vi "Write.vi"(5 "Maximum File Size (Bytes)":i64, 6 "Options":T1={"Delete All Excessive"=FALSE, "Delimiter"=",", "Enable Calendar Tree"=TRUE, "File Extension"="csv", "Time Stamp Format"="%Y%m%dT%H%M%S%3u"}, 7 "Maximum File Count":i32, 8 "Error In":errorcluster, 9 "Messages":T2[](array[typedef]), 10 "Bulk CSV Buffer In":string, 11 "Log In":refnum<file>) -> (0 "Error Out":errorcluster, 2 "Bulk CSV Buffer Out":string, 3 "Log Out":refnum<file>)   [LabVIEW 2025, in "LOGlib_LV2025.lvlib" / "File.lvlib"]
uses:
  File.lvlib
  Type Definitions/Statement.ctl
  Type Definitions/Tag.ctl
  Create ISO 8601 File Name.vi
  Write Header.vi
  Create Calendar Folder Tree.vi
  Get Oldest File.vi
  <vilib>/Utility/libraryn.llb/Check if File or Folder Exists.vi
  LOGlib_LV2025.lvlib
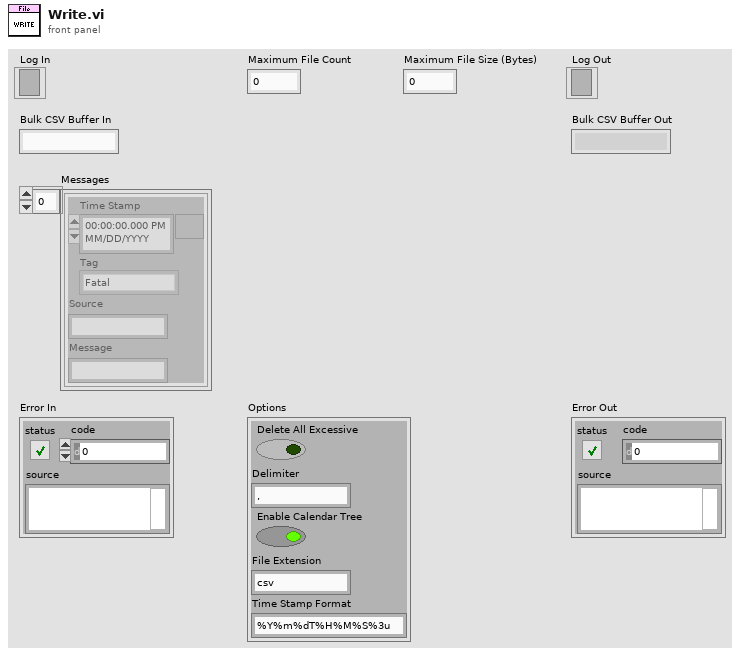
[diagram p1: front panel]
types:
  T1 = cluster{"Delete All Excessive":bool, "Delimiter":string, "Enable Calendar Tree":bool, "File Extension":string, "Time Stamp Format":string}
  T2 = typedef "LOGlib_LV2025.lvlib/Statement.ctl" = cluster{"Time Stamp":timestamp, "Tag":T3, "Source":string, "Message":string}
  T3 = typedef "LOGlib_LV2025.lvlib/Tag.ctl" = enum16{"Fatal", "Error", "Warn", "Info", "Debug", "Trace"}
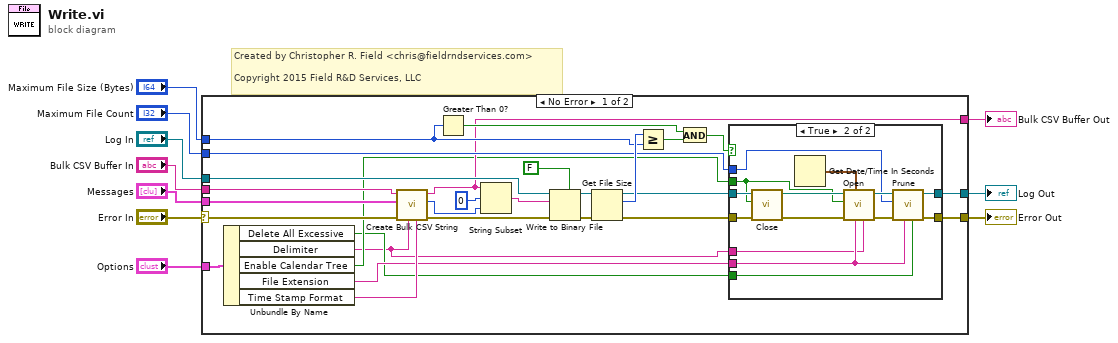
[diagram p0: block diagram]
diagram:
  # "Created by Christopher R. Field <chris@fieldrndservices.com>\n\nCopyright 2015 Field R&D Services, LLC"
  n1 = case shown="No Error" "Error In" {
    selector: "Error In" -> [w24 w56]
    tunnel: "Log In" -> [w38 w57]
    tunnel: "Messages" -> [w22 _]
    tunnel: [w28 w57] -> w7
    tunnel: [w27 w56] -> w6
    tunnel: "Maximum File Size (Bytes)" -> [w29 _]
    tunnel: "Maximum File Count" -> [w26 _]
    tunnel: "Bulk CSV Buffer In" -> [w21 w55]
    tunnel: [w17 w55] -> w2
    tunnel: "Options" -> [w16 _]
    frame No Error {
      n2 = Unbundle By Name(w16) -> ("Delete All Excessive"=w12:bool, "Delimiter"=w11:string, "Enable Calendar Tree"=w14:bool, "File Extension"=w13:string, "Time Stamp Format"=w15:string)
      n3 = call "Create Bulk CSV String.vi"("Time Stamp Format"=w15, "Delimiter"=w11, "Error In"=w24, "Messages"=w22, "Bulk CSV Buffer In"=w21) -> ("Error Out"=w23:errorcluster, "CSV Length"=w20:i32, "Bulk CSV Buffer Out"=w17:string)  [unwired: 4 in]
      n4 = Greater Than 0?(x=w29) -> (x > 0?=w36:bool)
      n5 = String Subset(string=w17, offset (0)=0, length (rest)=w20) -> (substring=w18:string)
      n6 = Write to Binary File(file (use dialog)=w38, data=w18, error in=w23, 5:FALSE ("prepend array or string size? (T)")) -> (refnum out=w31:refnum<file>, error out=w30:errorcluster)  [unwired: 2 in, 1 out]
      n7 = Get File Size(file=w31, error in=w30) -> (refnum out=w33:refnum<file>, size (in bytes)=w35:i64, 0:w32:errorcluster)
      n8 = Greater Or Equal?(x=w35, y=w29) -> (x >= y?=w37:bool)
      n9 = And(x=w36, y=w37) -> (x .and. y?=w34:bool)
      n10 = case shown="True" w34 {
        tunnel: [w40 w46] -> w28
        tunnel: [w39 w47] -> w27
        tunnel: w33 -> [w40 w53]
        tunnel: w32 -> [w39 w52]
        tunnel: w14 -> [_ w44]
        tunnel: w26 -> [_ w45]
        tunnel: w13 -> [_ w43]
        tunnel: w12 -> [_ w42]
        tunnel: w11 -> [_ w41]
        frame False {
        }
        frame True {
          n11 = call "Close.vi"("Error In"=w52, "Enable Calendar Tree"=w44, "Log In"=w53) -> ("Error Out"=w51:errorcluster, "Base Log Folder"=w50:path)  [unwired: 7 in]
          n12 = Get Date/Time In Seconds() -> (seconds since 1Jan1904=w54:timestamp)
          n13 = call "Open.vi"("Delimiter"=w41, "File Extension"=w43, "Start Time Stamp"=w54, "Error In"=w51, "Enable Calendar Tree"=w44, "Base Folder"=w50) -> ("Error Out"=w48:errorcluster, "Log Out"=w49:refnum<file>)  [unwired: 4 in]
          n14 = call "Prune.vi"("Delete All Excessive"=w42, "File Extension"=w43, "Error In"=w48, "Maximum File Count"=w45, "File In"=w49) -> ("Error Out"=w47:errorcluster, "File Out"=w46:refnum<file>)  [unwired: 5 in]
        }
      }
    }
    frame Error {
    }
  }
  "Log Out" <- w7
  "Error Out" <- w6
  "Bulk CSV Buffer Out" <- w2
